vi "Check_limits.vi"(0 "Distancia X/Y":i32, 5 "Tipo Movimiento":T1, 7 "Cluster_Tracking":T2, 9 "Distancia Z":i32, 11 "error in (no error)":errorcluster) -> (4 "Tipo Movimiento 2":T1, 6 "Cluster_Tracking 2":T2, 8 "Limite sobrepasado?":bool, 10 "Estado":T3, 15 "error out":errorcluster)   [LabVIEW 2019]
uses:
  Typedefs/Tipo_movimiento.ctl
  Typedefs/ESTADOS.ctl
  Typedefs/Cluster_tracking.ctl
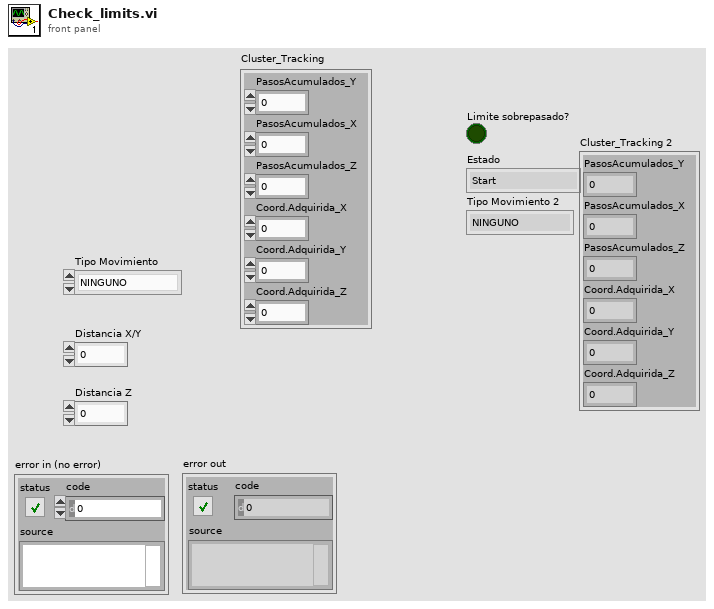
[diagram p1: front panel]
types:
  T1 = typedef "Tipo_movimiento.ctl" = enum16{"NINGUNO", "AVANZAR", "RETROCEDER", "DERECHA", "IZQUIERDA", "SUBIRZ", "BAJARZ", "HOME", "HOME_Z"}
  T2 = typedef "Cluster_tracking.ctl" = cluster{"PasosAcumulados_Y":i32, "PasosAcumulados_X":i32, "PasosAcumulados_Z":i32, "Coord.Adquirida_X":i32, "Coord.Adquirida_Y":i32, "Coord.Adquirida_Z":i32}
  T3 = typedef "ESTADOS.ctl" = enum16{"Start", "Ping_Arduino", "Init Refs", "Check Button", "Check Limits", "Home", "Cabezal Posicion Inicio", "Terminaste posicion inicio?", "Terminar", "Salir Arduino", "Envio Parametros Movimiento", "Recepcion Comando?", "Terminaste Movimiento?", "Adquirir Coordenada", "Terminaste Home?", "Salir"}
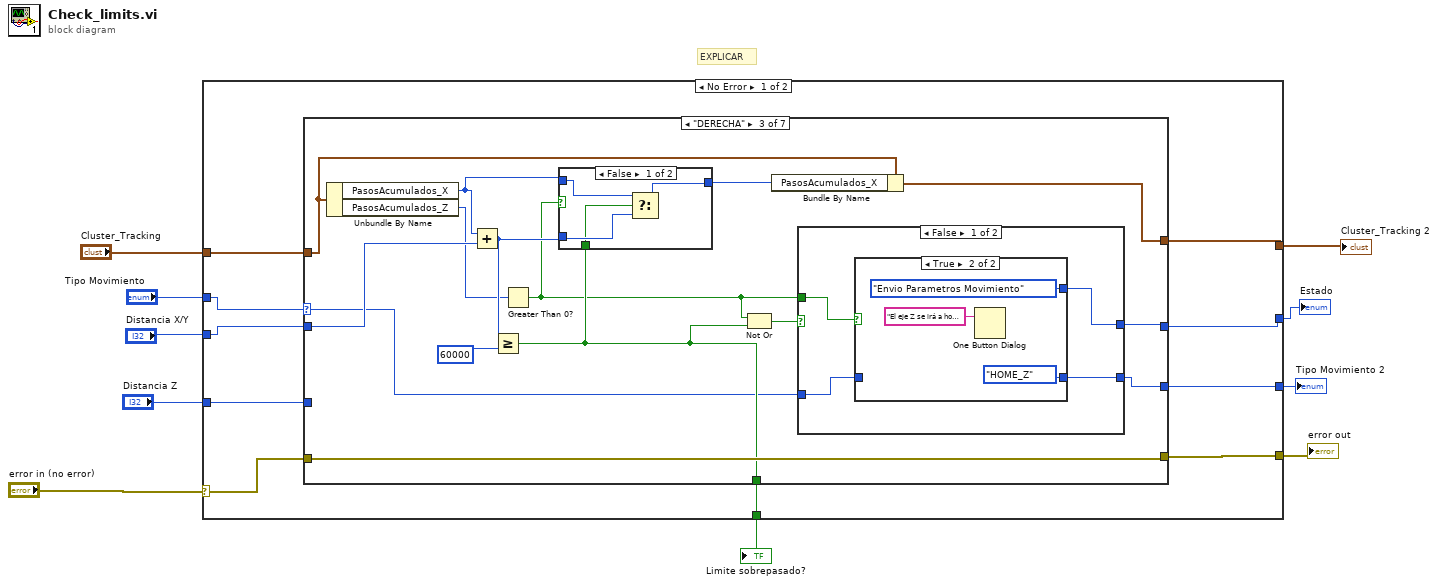
[diagram p0: block diagram]
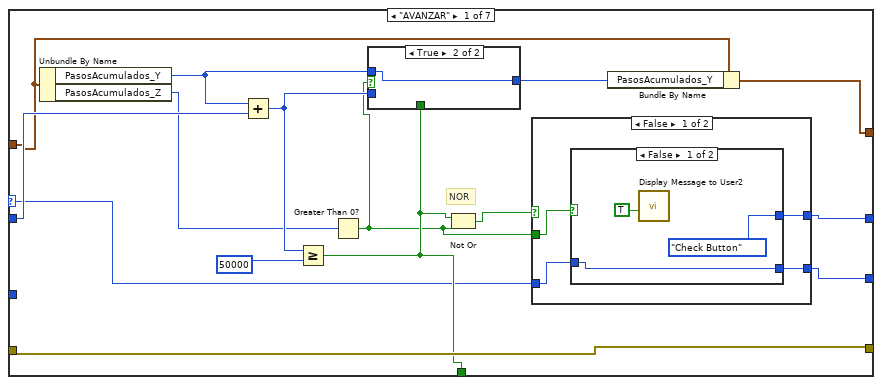
[diagram p2: hidden frame]
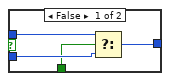
[diagram p3: hidden frame]
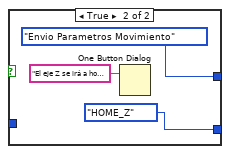
[diagram p4: hidden frame]
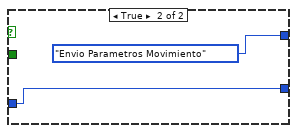
[diagram p5: hidden frame]
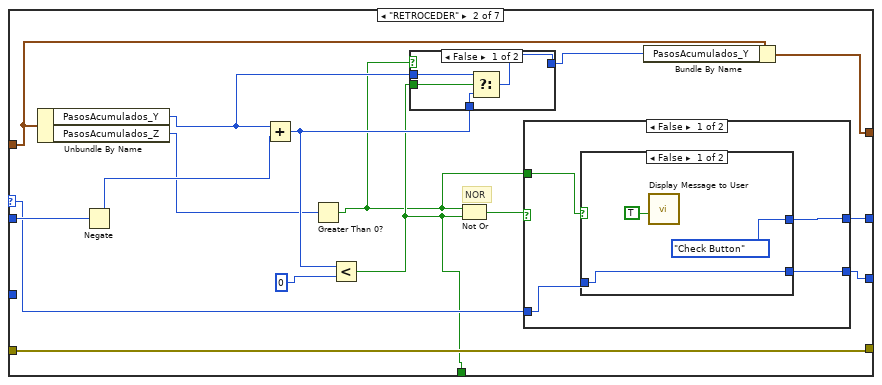
[diagram p6: hidden frame]
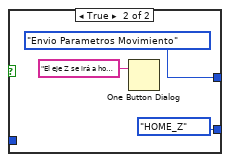
[diagram p8: hidden frame]
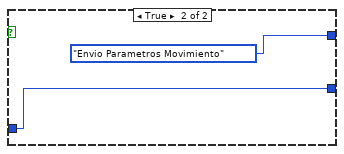
[diagram p9: hidden frame]
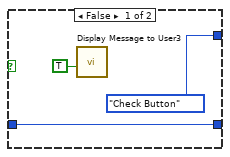
[diagram p11: hidden frame]
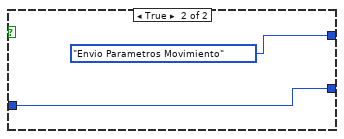
[diagram p12: hidden frame]
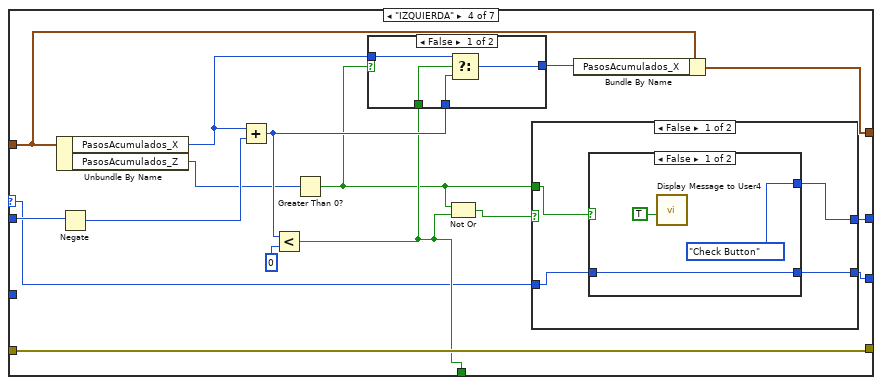
[diagram p13: hidden frame]
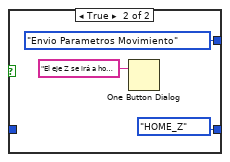
[diagram p15: hidden frame]
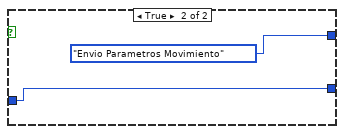
[diagram p16: hidden frame]
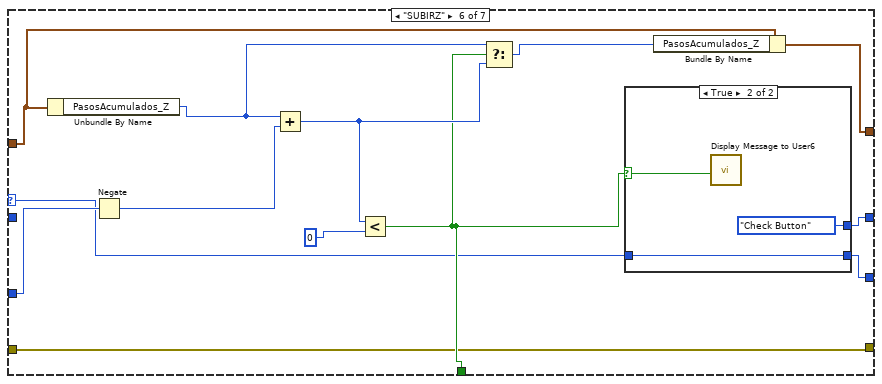
[diagram p18: hidden frame]
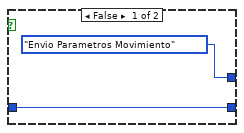
[diagram p19: hidden frame]
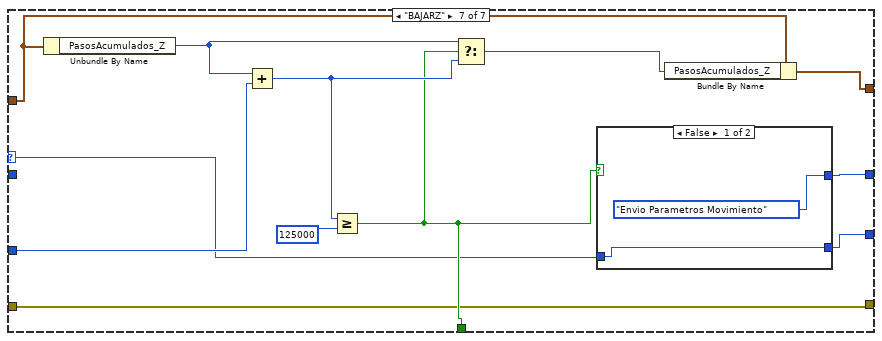
[diagram p20: hidden frame]
diagram:
  # "EXPLICAR"
  n1 = case shown="No Error" "error in (no error)" {
    selector: "error in (no error)" -> [w19 w191]
    tunnel: "Tipo Movimiento" -> [w20 w189]
    tunnel: "Distancia X/Y" -> [w17 _]
    tunnel: [w18 w191] -> w7
    tunnel: "Cluster_Tracking" -> [w16 w190]
    tunnel: [w15 w190] -> w5
    tunnel: [w14 _] -> w4
    tunnel: "Distancia Z" -> [w13 _]
    tunnel: [w12 _] -> w2
    tunnel: [w11 w189] -> w1
    frame No Error {
      n2 = case shown="\"DERECHA\"" w20 {
        selector: w20 -> [w24 w57 w89 w119 w151 w156 w173]
        tunnel: w17 -> [w33 w65 w98 w130 _ _ _]
        tunnel: [w31 w63 w96 w129 w153 w157 w175] -> w18
        tunnel: w19 -> [w31 w63 w96 w129 w153 w157 w175]
        tunnel: w16 -> [w28 w61 w94 w127 w152 w160 w179]
        tunnel: [w29 w60 w93 w125 w152 w159 w178] -> w15
        tunnel: [w27 w54 w91 w123 _ w158 w177] -> w14
        tunnel: w13 -> [_ _ _ _ _ w161 w176]
        tunnel: [w23 w55 w88 w120 _ w154 w174] -> w12
        tunnel: [w22 w56 w87 w121 w151 w155 w172] -> w11
        frame "AVANZAR" {
          # "NOR"
          n3 = Unbundle By Name(w28) -> ("PasosAcumulados_Y"=w32:i32, "PasosAcumulados_Z"=w26:i32)
          n4 = Add(x=w32, y=w33) -> (x+y=w34:i32)
          n5 = Greater Or Equal?(x=w34, y=50000) -> (x >= y?=w27:bool)
          n6 = Greater Than 0?(x=w26) -> (x > 0?=w21:bool)
          n7 = case shown="True" w21 {
            tunnel: w34 -> [w39 _]
            tunnel: w32 -> [w38 w40]
            tunnel: [w37 w40] -> w30
            tunnel: w27 -> [w36 _]
            frame False {
              n8 = Select(t=w38, s=w36, f=w39) -> (s? t:f=w37:i32)
            }
            frame True {
            }
          }
          n9 = Not Or(1:w21, 2:w27) -> (0:w25:bool)
          n10 = case shown="False" w25 {
            tunnel: [w43 ESTADOS."Envio Parametros Movimiento" ("Enum")] -> w23
            tunnel: w21 -> [w44 _]
            tunnel: [w42 w51] -> w22
            tunnel: w24 -> [w41 w51]
            frame False {
              n11 = case shown="False" w44 {
                tunnel: [ESTADOS."Check Button" ("Enum") ESTADOS."Envio Parametros Movimiento" ("Enum")] -> w43
                tunnel: [w46 Tipo_movimiento."HOME_Z" ("Tipo Movimiento 2")] -> w42
                tunnel: w41 -> [w46 _]
                frame False {
                  n12 = call "Display Message to User2"("Enable"=TRUE) -> ()  [unwired: 9 in, 2 out]
                }
                frame True {
                  n13 = One Button Dialog(message="El eje Z se irá a home por seguridad para continuar el desplazamiento en X o Y.") -> ()  [unwired: 1 in, 1 out]
                }
              }
            }
            frame True {
            }
          }
          n14 = Bundle By Name(cluster=w28, "PasosAcumulados_Y"=w30) -> (w29:T2)
        }
        frame "RETROCEDER" {
          # "NOR"
          n15 = Unbundle By Name(w61) -> ("PasosAcumulados_Y"=w64:i32, "PasosAcumulados_Z"=w59:i32)
          n16 = Negate(x=w65) -> (-x=w68:i32)
          n17 = Add(x=w64, y=w68) -> (x+y=w66:i32)
          n18 = Greater Than 0?(x=w59) -> (x > 0?=w53:bool)
          n19 = Less?(x=w66, y=0) -> (x < y?=w54:bool)
          n20 = case shown="False" w53 {
            tunnel: w66 -> [w72 _]
            tunnel: w64 -> [w71 w73]
            tunnel: [w70 w73] -> w62
            tunnel: w54 -> [w69 _]
            frame False {
              n21 = Select(t=w71, s=w69, f=w72) -> (s? t:f=w70:i32)
            }
            frame True {
            }
          }
          n22 = Not Or(1:w54, 2:w53) -> (0:w58:bool)
          n23 = case shown="False" w58 {
            tunnel: [w77 ESTADOS."Envio Parametros Movimiento" ("Enum")] -> w55
            tunnel: [w76 w84] -> w56
            tunnel: w53 -> [w75 _]
            tunnel: w57 -> [w74 w84]
            frame False {
              n24 = case shown="False" w75 {
                tunnel: [ESTADOS."Check Button" ("Enum") ESTADOS."Envio Parametros Movimiento" ("Enum")] -> w77
                tunnel: [w78 Tipo_movimiento."HOME_Z" ("Tipo Movimiento 2")] -> w76
                tunnel: w74 -> [w78 _]
                frame False {
                  n25 = call "Display Message to User"("Enable"=TRUE) -> ()  [unwired: 9 in, 2 out]
                }
                frame True {
                  n26 = One Button Dialog(message="El eje Z se irá a home por seguridad para continuar el desplazamiento en X o Y.") -> ()  [unwired: 1 in, 1 out]
                }
              }
            }
            frame True {
            }
          }
          n27 = Bundle By Name(cluster=w61, "PasosAcumulados_Y"=w62) -> (w60:T2)
        }
        frame "DERECHA" {
          n28 = Unbundle By Name(w94) -> ("PasosAcumulados_X"=w97:i32, "PasosAcumulados_Z"=w92:i32)
          n29 = Add(x=w97, y=w98) -> (x+y=w99:i32)
          n30 = Greater Or Equal?(x=w99, y=60000) -> (x >= y?=w91:bool)
          n31 = Greater Than 0?(x=w92) -> (x > 0?=w86:bool)
          n32 = case shown="False" w86 {
            tunnel: w99 -> [w104 _]
            tunnel: w97 -> [w103 w105]
            tunnel: [w102 w105] -> w95
            tunnel: w91 -> [w101 _]
            frame False {
              n33 = Select(t=w103, s=w101, f=w104) -> (s? t:f=w102:i32)
            }
            frame True {
            }
          }
          n34 = Not Or(1:w91, 2:w86) -> (0:w90:bool)
          n35 = Bundle By Name(cluster=w94, "PasosAcumulados_X"=w95) -> (w93:T2)
          n36 = case shown="False" w90 {
            tunnel: [w109 ESTADOS."Envio Parametros Movimiento" ("Enum")] -> w88
            tunnel: [w108 w116] -> w87
            tunnel: w89 -> [w106 w116]
            tunnel: w86 -> [w107 _]
            frame False {
              n37 = case shown="True" w107 {
                tunnel: [ESTADOS."Check Button" ("Enum") ESTADOS."Envio Parametros Movimiento" ("Enum")] -> w109
                tunnel: [w110 Tipo_movimiento."HOME_Z" ("Tipo Movimiento 2")] -> w108
                tunnel: w106 -> [w110 _]
                frame False {
                  n38 = call "Display Message to User3"("Enable"=TRUE) -> ()  [unwired: 9 in, 2 out]
                }
                frame True {
                  n39 = One Button Dialog(message="El eje Z se irá a home por seguridad para continuar el desplazamiento en X o Y.") -> ()  [unwired: 1 in, 1 out]
                }
              }
            }
            frame True {
            }
          }
        }
        frame "IZQUIERDA" {
          n40 = Unbundle By Name(w127) -> ("PasosAcumulados_X"=w128:i32, "PasosAcumulados_Z"=w124:i32)
          n41 = Negate(x=w130) -> (-x=w133:i32)
          n42 = Add(x=w128, y=w133) -> (x+y=w131:i32)
          n43 = Less?(x=w131, y=0) -> (x < y?=w123:bool)
          n44 = Greater Than 0?(x=w124) -> (x > 0?=w118:bool)
          n45 = case shown="False" w118 {
            tunnel: w131 -> [w137 _]
            tunnel: w128 -> [w136 w138]
            tunnel: [w135 w138] -> w126
            tunnel: w123 -> [w134 _]
            frame False {
              n46 = Select(t=w136, s=w134, f=w137) -> (s? t:f=w135:i32)
            }
            frame True {
            }
          }
          n47 = Not Or(1:w123, 2:w118) -> (0:w122:bool)
          n48 = case shown="False" w122 {
            tunnel: [w142 ESTADOS."Envio Parametros Movimiento" ("Enum")] -> w120
            tunnel: [w141 w149] -> w121
            tunnel: w118 -> [w140 _]
            tunnel: w119 -> [w139 w149]
            frame False {
              n49 = case shown="False" w140 {
                tunnel: [ESTADOS."Check Button" ("Enum") ESTADOS."Envio Parametros Movimiento" ("Enum")] -> w142
                tunnel: [w143 Tipo_movimiento."HOME_Z" ("Tipo Movimiento 2")] -> w141
                tunnel: w139 -> [w143 _]
                frame False {
                  n50 = call "Display Message to User4"("Enable"=TRUE) -> ()  [unwired: 9 in, 2 out]
                }
                frame True {
                  n51 = One Button Dialog(message="El eje Z se irá a home por seguridad para continuar el desplazamiento en X o Y.") -> ()  [unwired: 1 in, 1 out]
                }
              }
            }
            frame True {
            }
          }
          n52 = Bundle By Name(cluster=w127, "PasosAcumulados_X"=w126) -> (w125:T2)
        }
        frame "NINGUNO", Default {
        }
        frame "SUBIRZ" {
          n53 = Unbundle By Name(w160) -> ("PasosAcumulados_Z"=w163:i32)
          n54 = Negate(x=w161) -> (-x=w166:i32)
          n55 = Add(x=w163, y=w166) -> (x+y=w164:i32)
          n56 = Less?(x=w164, y=0) -> (x < y?=w158:bool)
          n57 = Select(t=w163, s=w158, f=w164) -> (s? t:f=w162:i32)
          n58 = case shown="True" w158 {
            selector: w158 -> [_ w171]
            tunnel: [ESTADOS."Envio Parametros Movimiento" ("Enum") ESTADOS."Check Button" ("Enum")] -> w154
            tunnel: w156 -> [w167 w169]
            tunnel: [w167 w169] -> w155
            frame False {
            }
            frame True {
              n59 = call "Display Message to User6"("Enable"=w171) -> ()  [unwired: 9 in, 2 out]
            }
          }
          n60 = Bundle By Name(cluster=w160, "PasosAcumulados_Z"=w162) -> (w159:T2)
        }
        frame "BAJARZ" {
          n61 = Unbundle By Name(w179) -> ("PasosAcumulados_Z"=w181:i32)
          n62 = Add(x=w181, y=w176) -> (x+y=w182:i32)
          n63 = Greater Or Equal?(x=w182, y=125000) -> (x >= y?=w177:bool)
          n64 = Select(t=w181, s=w177, f=w182) -> (s? t:f=w180:i32)
          n65 = case shown="False" w177 {
            selector: w177 -> [_ w188]
            tunnel: [ESTADOS."Envio Parametros Movimiento" ("Enum") ESTADOS."Check Button" ("Enum")] -> w174
            tunnel: [w184 w186] -> w172
            tunnel: w173 -> [w184 w186]
            frame False {
            }
            frame True {
              n66 = call "Display Message to User5"("Enable"=w188) -> ()  [unwired: 9 in, 2 out]
            }
          }
          n67 = Bundle By Name(cluster=w179, "PasosAcumulados_Z"=w180) -> (w178:T2)
        }
      }
    }
    frame Error {
    }
  }
  "error out" <- w7
  "Estado" <- w2
  "Cluster_Tracking 2" <- w5
  "Limite sobrepasado?" <- w4
  "Tipo Movimiento 2" <- w1
